vi "Wait for Acquisition Complete.vi"(8 "error in (no error)":errorcluster, 9 "Maximum Time (10000)":u32=10000, 11 "VISA resource name":refnum<visa-resource-name>) -> (0 "error out":errorcluster, 3 "VISA resource name out":refnum<visa-resource-name>)   [LabVIEW 2011, in "Template - Spectrum Analyzer.lvlib"]
doc: "Waits for the current sweep to finish. This VI should be called after Initiate VI and before Fetch Trace VI.\n\n<B>Note:</B> \n\nUse this VI only with other low-level VIs. The high-level VIs automatically incorporate this functionality. This VI does not check the instrument status."
uses:
  <instrlib>/_Template - Spectrum Analyzer/Template - Spectrum Analyzer.lvlib
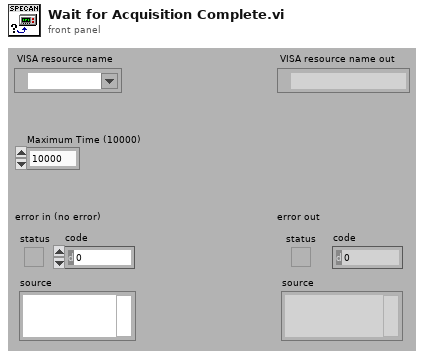
[diagram p1: front panel]
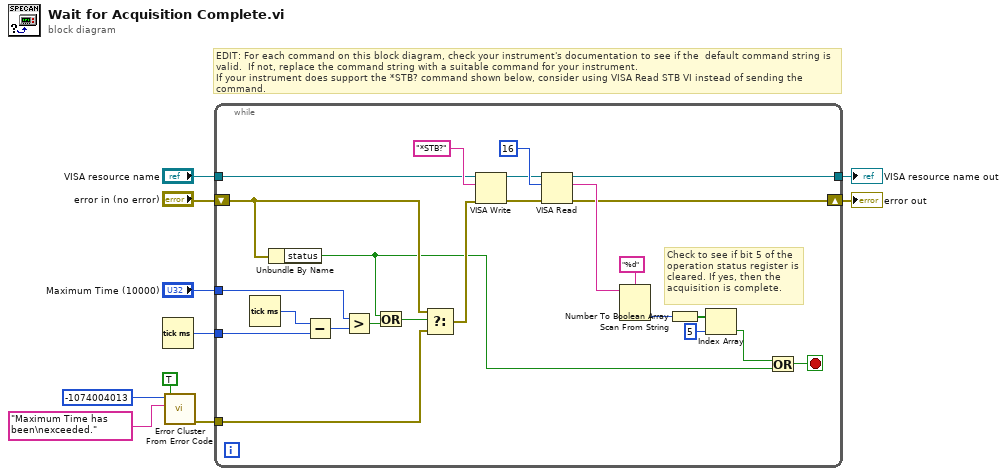
[diagram p0: block diagram]
diagram:
  # "EDIT: For each command on this block diagram, check your instrument's documentation to see if the  default command string is valid.  If not, replace the command string with a suitable command for your instrument. \nIf your instrument does support the *STB? command shown below, consider using VISA Read STB VI instead of sending the command."
  n1 = Tick Count (ms)() -> (millisecond timer value=w5:u32)
  n2 = call <vilib>:"Error Cluster From Error Code.vi"("show call chain? (False)"=TRUE, "error message (\"\")"="Maximum Time has been\nexceeded." ("error message (\"\")"), "error code (0)"=-1074004013) -> ("error out"=w1:errorcluster)  [unwired: 6 in]
  n3 = while {
    tunnel: [w31] -> w9
    tunnel: "VISA resource name" -> [w28]
    tunnel: "Maximum Time (10000)" -> [w22]
    tunnel: w5 -> [w23]
    shift-right: [w32] -> w10
    shift-left: "error in (no error)" -> [w14]
    tunnel: w1 -> [w12]
    stop <- w18 stop-if-true
    # "Check to see if bit 5 of the operation status register is cleared. If yes, then the acquisition is complete."
    n4 = Tick Count (ms)() -> (millisecond timer value=w25:u32)
    n5 = Unbundle By Name(w14) -> ("status"=w11:bool)
    n6 = Subtract(x=w25, y=w23) -> (x-y=w24:u32)
    n7 = Greater?(x=w22, y=w24) -> (0:w15:bool)
    n8 = Or(x=w11, y=w15) -> (x .or. y?=w16:bool)
    n9 = Select(t=w14, s=w16, f=w12) -> (s? t:f=w13:errorcluster)
    n10 = VISA Write(VISA resource name=w28, write buffer="*STB?", error in (no error)=w13) -> (VISA resource name out=w26:refnum<visa-resource-name>, error out=w27:errorcluster)  [unwired: 1 out]
    n11 = VISA Read(VISA resource name=w26, byte count=u32 16, error in (no error)=w27) -> (VISA resource name out=w31:refnum<visa-resource-name>, read buffer=w34:string, error out=w32:errorcluster)  [unwired: 1 out]
    n12 = Scan From String(format string="%d", input string=w34) -> (output 1=w20:i32)  [unwired: 3 in, 3 out]
    n13 = Number To Boolean Array(number=w20) -> (Boolean array=w19:bool[])
    n14 = Index Array(array=w19, index=5) -> (element=w17:bool)
    n15 = Or(x=w17, y=w11) -> (x .or. y?=w18:bool)
  }
  "error out" <- w10
  "VISA resource name out" <- w9
